vi "SLL Easy API Client Write Example.vi"() -> ()   [LabVIEW 2016, in "SLL Easy API via TCP.lvclass"]
uses:
  SLL Easy API via TCP.lvclass
  _SubVIs/TCP Initialize Client - Local.vi
panel:
  out "error out":errorcluster
  in  "Write Data":string="Sample Write Data"
  in  "Service Name":string="SLL Easy TCP Service"
  # "Run the Server VI Example before running this VI"
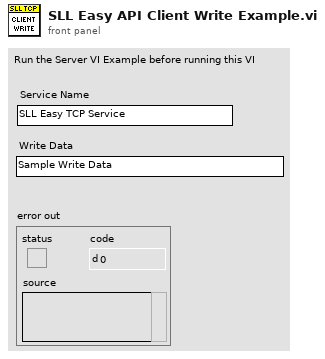
[diagram p1: front panel]
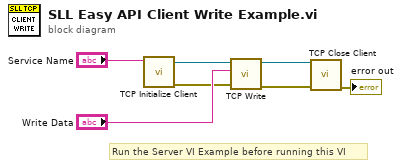
[diagram p0: block diagram]
diagram:
  # "Run the Server VI Example before running this VI"
  n1 = call-poly "TCP Initialize Client.vi"("Service Name"="Service Name") -> ("error out"=w3:errorcluster, "connection ID Out"=w7:refnum<k5>)  [unwired: 9 in]
  n2 = call "TCP Write.vi"("error in (no error)"=w3, "Write Data"="Write Data", "connection ID In"=w7) -> ("error out"=w2:errorcluster, "connection ID Out"=w6:refnum<k5>)  [unwired: 7 in]
  n3 = call "TCP Close Client.vi"("error in (no error)"=w2, "connection ID"=w6) -> ("error out"=→"error out":errorcluster)  [unwired: 9 in]
